vi "Configure All.vi"(1 "RT Data in":T1={"Device ref"=0, "Scan Period (uSec)"=10000, "Device Channels"={"Status"={"BD Refs"=[], "Length"=0, "FIFO Index"=0, "Data"=[]}, "Command"={"BD Refs"=[], "Data"=[], "Length"=0, "FIFO Index"=0}}, "Local Chassis"=[], "EtherCAT Masters"=[], "Async"={"Status"=refnum, "Command"=refnum, "Input FIFO"=refnum, "Input FIFO buffer"=[], "Output FIFO"=refnum, "Output FIFO buffer"=[], "Async VI Ref"=refnum}, "ECAT Reconfig"={"Reconfig Module Found"=FALSE, "VI Ref"=refnum, "Status"=refnum}, "Device Error"={"status"=FALSE, "code"=0, "source"=""}, "DeviceName"="", "PCLSync?"=FALSE} {"Device Channels"."Status"."BD Refs"."Data Reference" format="%.0x"; "Device Channels"."Command"."BD Refs"."Data Reference" format="%.0x"; "Local Chassis"."FPGA"."VS ref" format="%.0x"; "Local Chassis"."RSI Modules"."VS ref" format="%.0x"; "Local Chassis"."VS ref" format="%.0x"; "Device ref" format="%.0x"; "EtherCAT Masters"."REM IO ECAT Slaves"."VS ref" format="%.0x"; "EtherCAT Masters"."Generic EtherCAT Slaves"."VS ref" format="%.0x"; "EtherCAT Masters"."VS ref" format="%.0x"; "EtherCAT Masters"."EtherCAT Slaves"."FPGA"."VS ref" format="%.0x"; "EtherCAT Masters"."EtherCAT Slaves"."RSI Modules"."VS ref" format="%.0x"; "EtherCAT Masters"."EtherCAT Slaves"."VS ref" format="%.0x"}) -> (0 "RT Data out":T1={"Device ref"=0, "Scan Period (uSec)"=10000, "Device Channels"={"Status"={"BD Refs"=[], "Length"=0, "FIFO Index"=0, "Data"=[]}, "Command"={"BD Refs"=[], "Data"=[], "Length"=0, "FIFO Index"=0}}, "Local Chassis"=[], "EtherCAT Masters"=[], "Async"={"Status"=refnum, "Command"=refnum, "Input FIFO"=refnum, "Input FIFO buffer"=[], "Output FIFO"=refnum, "Output FIFO buffer"=[], "Async VI Ref"=refnum}, "ECAT Reconfig"={"Reconfig Module Found"=FALSE, "VI Ref"=refnum, "Status"=refnum}, "Device Error"={"status"=FALSE, "code"=0, "source"=""}, "DeviceName"="", "PCLSync?"=FALSE} {"Device Channels"."Status"."BD Refs"."Data Reference" format="%.0x"; "Device Channels"."Command"."BD Refs"."Data Reference" format="%.0x"; "Local Chassis"."FPGA"."VS ref" format="%.0x"; "Local Chassis"."RSI Modules"."VS ref" format="%.0x"; "Local Chassis"."VS ref" format="%.0x"; "Device ref" format="%.0x"; "EtherCAT Masters"."REM IO ECAT Slaves"."VS ref" format="%.0x"; "EtherCAT Masters"."Generic EtherCAT Slaves"."VS ref" format="%.0x"; "EtherCAT Masters"."VS ref" format="%.0x"; "EtherCAT Masters"."EtherCAT Slaves"."FPGA"."VS ref" format="%.0x"; "EtherCAT Masters"."EtherCAT Slaves"."RSI Modules"."VS ref" format="%.0x"; "EtherCAT Masters"."EtherCAT Slaves"."VS ref" format="%.0x"})   [LabVIEW 2020, in "SEECD Engine.lvlib"]
uses:
  SEECD Engine.lvlib
  Type Defs/RT Data.ctl
  <vilib>/NI VeriStand/Custom Device API/Custom Device Item Ref.ctl
  Type Defs/Device Channels.ctl
  Type Defs/Output Data.ctl
  <vilib>/NI VeriStand/Custom Device API/Block Data Reference.ctl
  <vilib>/NI VeriStand/Custom Device API/Data Reference.ctl
  Type Defs/Input Data.ctl
  Type Defs/Local Chassis Data.ctl
  Type Defs/RSI Module Data.ctl
  Type Defs/Open Module IOVs.ctl
  Includes/Modules.lvlibp/RSI Module/RSI Module.lvclass
  Includes/Modules.lvlibp/RSI Module/Module Models.ctl
  Includes/Modules.lvlibp/RSI Module/Channel Type.ctl
  Type Defs/Module Config Data.ctl
  Type Defs/Mixed IO.ctl
  Type Defs/FPGA Data.ctl
  Type Defs/UDV Data.ctl
  Shared/Type Defs/UDV Data Type.ctl
  Shared/Type Defs/FXP Config.ctl
  Type Defs/Mod Size Indexes.ctl
  Type Defs/EtherCAT Master Data.ctl
  Type Defs/EtherCAT Slave Data.ctl
  Type Defs/Generic ECAT Slave RT-Data-Array.ctl
  Type Defs/Generic ECAT Slave Data Cluster.ctl
  Type Defs/Generic ECAT Slave IOV Cluster.ctl
  Type Defs/REM IO ECAT Slave RT-Data-Array.ctl
  Type Defs/REM IO ECAT Slave Data Cluster.ctl
  Type Defs/REM IO ECAT Slave IOV Cluster.ctl
  Type Defs/Async Data.ctl
  Type Defs/Async Status.ctl
  Type Defs/Async State.ctl
  Type Defs/Async Command.ctl
  Type Defs/ECAT Reconfig Data.ctl
  Type Defs/ECAT Reconfig Status.ctl
  Type Defs/ECAT Reconfig State.ctl
  Type Defs/ECAT Module Reconfig.ctl
  <vilib>/NI VeriStand/Custom Device Tools/Custom Device Utility Library/Custom Device Utility Library.lvlib
  <resource>/objmgr/IndComECAT.rc
  <vilib>/NI VeriStand/Custom Device API/Custom Device API.lvlib
  Shared/SEECD Shared.lvlib
types:
  T1 = typedef "SEECD Engine.lvlib/RT Data.ctl" = cluster{"Device ref":T2, "Scan Period (uSec)":u32, "Device Channels":T3, "Local Chassis":T8[], "EtherCAT Masters":T20[], "Async":T28, "ECAT Reconfig":T29, "Device Error":errorcluster, "DeviceName":string, "PCLSync?":bool}
  T2 = typedef "Custom Device API.lvlib/Custom Device Item Ref.ctl" = u64
  T3 = typedef "SEECD Engine.lvlib/Device Channels.ctl" = cluster{"Status":T4, "Command":T7}
  T4 = typedef "SEECD Engine.lvlib/Output Data.ctl" = cluster{"BD Refs":T5[], "Length":i32, "FIFO Index":i32, "Data":dbl[]}
  T5 = typedef "Custom Device API.lvlib/Block Data Reference.ctl" = cluster{"Data Reference":T6, "Offset":u64, "Length":u64}
  T6 = typedef "Custom Device API.lvlib/Data Reference.ctl" = i32
  T7 = typedef "SEECD Engine.lvlib/Input Data.ctl" = cluster{"BD Refs":T5[], "Data":dbl[], "Length":i32, "FIFO Index":i32}
  T8 = typedef "SEECD Engine.lvlib/Local Chassis Data.ctl" = cluster{"VS ref":T2, "RSI Modules":T9[], "FPGA":T15[], "Input Mod Size Idxs":T19, "Output Modules":i32[], "MixedIO Mod Size Idxs":T19}
  T9 = typedef "SEECD Engine.lvlib/RSI Module Data.ctl" = cluster{"VS ref":T2, "IOV ref":refnum<k21>, "Open Mod refs":T10, "Module DVR":refnum<data-value>, "Slot":u32, "Model":T11, "Channel Type":T12, "EtherCAT?":bool, "CDInput Data":T7, "CDOutput Data":T4, "Module Config Data":T13, "Mixed IO":T14}
  T10 = typedef "SEECD Engine.lvlib/Open Module IOVs.ctl" = cluster{"Analog Read":refnum<k21>, "Digital Read":refnum<k21>, "Analog Write":refnum<k21>, "Digital Write":refnum<k21>}
  T11 = typedef "Modules.lvlibp/RSI Module.lvclass/Module Models.ctl" = enum16{"Empty", "NI 9201", "NI 9203", "NI 9205", "NI 9206", "NI 9207", "NI 9208", "NI 9209", "NI 9210", "NI 9211", "NI 9212", "NI 9213", "NI 9214", "NI 9215", "NI 9216", "NI 9217", "NI 9219", "NI 9220", "NI 9221", "NI 9222", "NI 9223", "NI 9224", "NI 9225", "NI 9226", "NI 9227", "NI 9228", "NI 9229", "NI 9233", "NI 9234", "NI 9235", "NI 9236", "NI 9237", "NI 9239", "NI 9242", "NI 9244", "NI 9253", "NI 9263", "NI 9264", "NI 9265", "NI 9266", "NI 9269", "NI 9344", "NI 9350", "NI 9375", "NI 9401", "NI 9402", "NI 9403", "NI 9411", "NI 9421", "NI 9422", "NI 9423", "NI 9425", "NI 9426", "NI 9435", "NI 9436", "NI 9437", "NI 9472", "NI 9474", "NI 9475", "NI 9476", "NI 9477", "NI 9478", "NI 9481", "NI 9482", "NI 9485"}
  T12 = typedef "Modules.lvlibp/RSI Module.lvclass/Channel Type.ctl" = enum16{"Analog", "Digital"}
  T13 = typedef "SEECD Engine.lvlib/Module Config Data.ctl" = cluster{"Configurable?":bool, "Config Block Data Refs":T5[], "Config Data DVR":refnum<data-value>, "Previous Values":dbl[], "Local Reconfig VI Ref":refnum<vi>}
  T14 = typedef "SEECD Engine.lvlib/Mixed IO.ctl" = cluster{"Input Channel Indices":i32[], "Input Buffer":dbl[]}
  T15 = typedef "SEECD Engine.lvlib/FPGA Data.ctl" = cluster{"VS ref":T2, "IOV ref":refnum<k21>, "FPGA Target":enum16{"Local", "EtherCAT"}, "Product Code":u32, "Bitfile Signature":string, "Bitfile Path (RT)":path, "FPGA Session":u32, "Input Data":T7, "Output Data":T4, "UDVs":cluster{"From FPGA":T16[], "To FPGA":T16[]}}
  T16 = typedef "SEECD Engine.lvlib/UDV Data.ctl" = cluster{"VS ref":T2, "IOV Ref":refnum<k21>, "Name":string, "UDV Data Type":T17, "Supported Type?":bool, "FXP Config":T18, "FXP VI Ref":refnum<vi>}
  T17 = typedef "SEECD Shared.lvlib/UDV Data Type.ctl" = enum16{"Boolean", "Fixed Point", "Int8", "Int16", "Int32", "Int64", "U32 Bit Field", "UInt8", "UInt16", "UInt32", "UInt64", "Other", "DBL", "SGL"}
  T18 = typedef "SEECD Shared.lvlib/FXP Config.ctl" = cluster{"signed":bool, "size":u32, "integersize":i32}
  T19 = typedef "SEECD Engine.lvlib/Mod Size Indexes.ctl" = cluster{"4":i32[], "8":i32[], "16":i32[], "32":i32[], "other":i32[]}
  T20 = typedef "SEECD Engine.lvlib/EtherCAT Master Data.ctl" = cluster{"VS ref":T2, "IOV ref":refnum<k21>, "Master ID":u32, "Cyclic Data Bandwidth":u32, "EtherCAT Slaves":T21[], "Generic EtherCAT Slaves":T22, "REM IO ECAT Slaves":T25}
  T21 = typedef "SEECD Engine.lvlib/EtherCAT Slave Data.ctl" = cluster{"VS ref":T2, "IOV ref":refnum<k21>, "Position Address":u16, "RSI Modules":T9[], "FPGA":T15[], "Input Mod Size Idxs":T19, "Output Modules":i32[], "MixedIO Mod Size Idxs":T19}
  T22 = typedef "SEECD Engine.lvlib/Generic ECAT Slave RT-Data-Array.ctl" = T23[]
  T23 = typedef "SEECD Engine.lvlib/Generic ECAT Slave Data Cluster.ctl" = cluster{"VS ref":T2, "IOV ref":refnum<k21>, "Position Address":u16, "I/O Imput Vars ":T24[], "I/O Output Vars":T24[], "I/O Input Data":T7, "I/O Output Data":T4, "Distributed Clock":bool}
  T24 = typedef "SEECD Engine.lvlib/Generic ECAT Slave IOV Cluster.ctl" = cluster{"VS ref":T2, "IOV Ref":refnum<k21>, "Name":string, "UDV Data Type":T17}
  T25 = typedef "SEECD Engine.lvlib/REM IO ECAT Slave RT-Data-Array.ctl" = T26[]
  T26 = typedef "SEECD Engine.lvlib/REM IO ECAT Slave Data Cluster.ctl" = cluster{"VS ref":T2, "IOV ref":refnum<k21>, "Position Address":u16, "I/O Imput Vars ":T27[], "I/O Output Vars":T27[], "I/O Input Data":T7, "I/O Output Data":T4}
  T27 = typedef "SEECD Engine.lvlib/REM IO ECAT Slave IOV Cluster.ctl" = cluster{"VS ref":T2, "IOV Ref":refnum<k21>, "Name":string, "UDV Data Type":T17, "Scaling Factor":dbl}
  T28 = typedef "SEECD Engine.lvlib/Async Data.ctl" = cluster{"Status":refnum<queue>, "Command":refnum<queue>, "Input FIFO":refnum<k33>, "Input FIFO buffer":dbl[], "Output FIFO":refnum<k33>, "Output FIFO buffer":dbl[], "Async VI Ref":refnum<vi>}
  T29 = typedef "SEECD Engine.lvlib/ECAT Reconfig Data.ctl" = cluster{"Reconfig Module Found":bool, "VI Ref":refnum<vi>, "Status":refnum<queue>}
  T30 = typedef "SEECD Engine.lvlib/ECAT Module Reconfig.ctl" = cluster{"Module DVR":refnum<data-value>, "IOV ref":refnum<k21>, "Config Data DVR":refnum<data-value>}
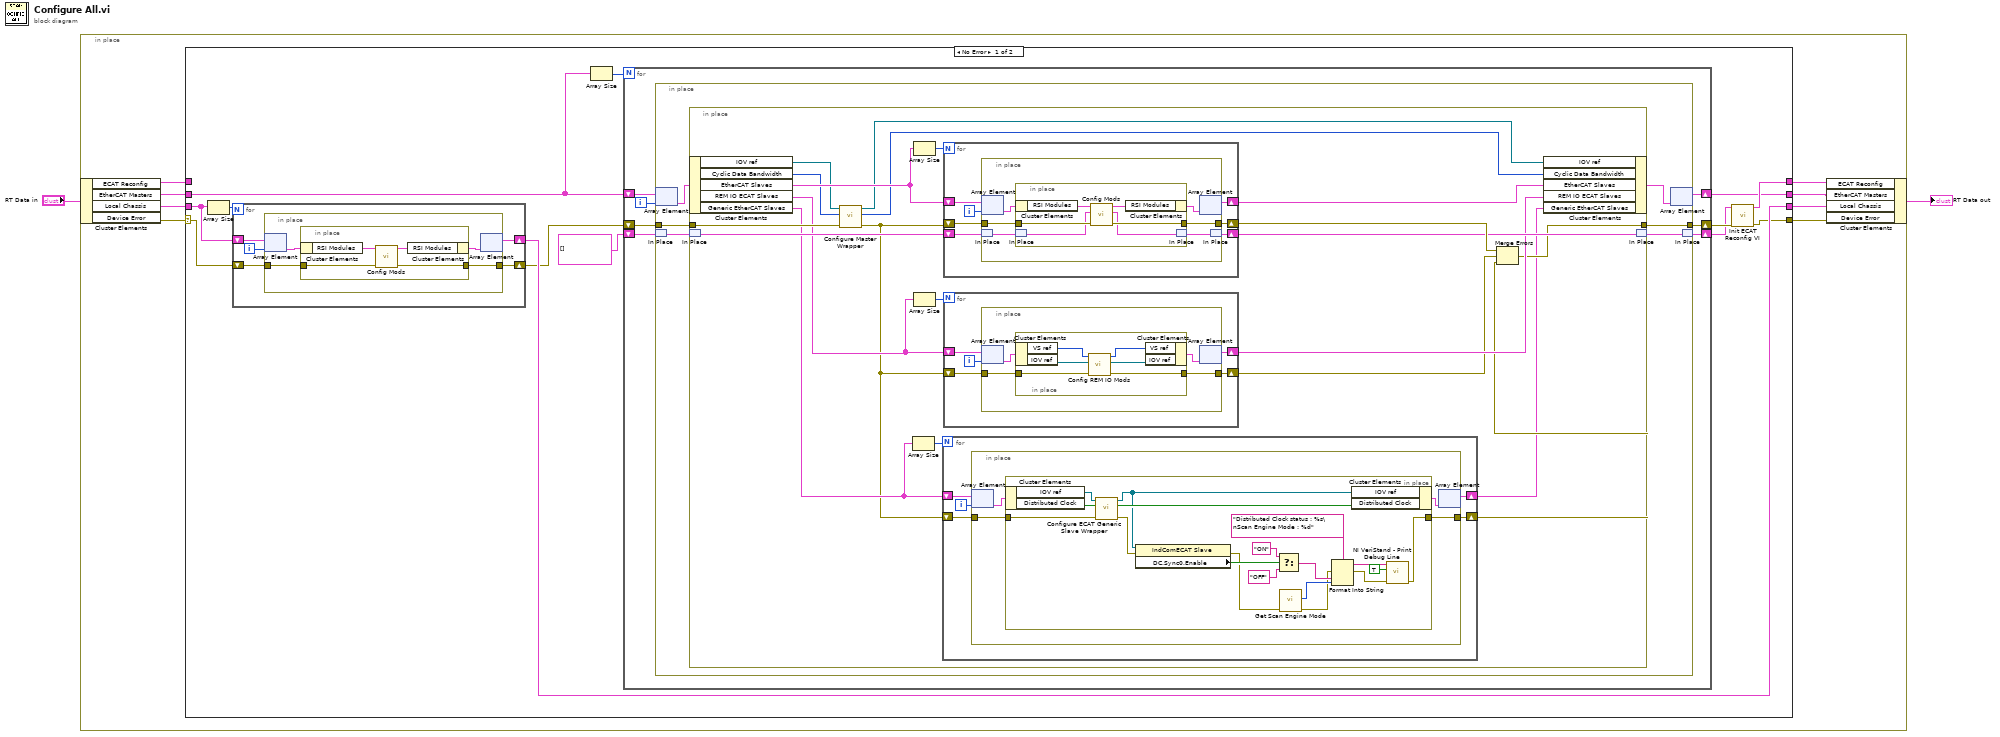
[diagram p0: block diagram]
diagram:
  n1 = in-place {
    n2 = in-place-cluster #1("RT Data in") -> ("ECAT Reconfig"=w3:T29, "EtherCAT Masters"=w9:T20[], "Local Chassis"=w8:T8[], "Device Error"=w10:errorcluster)
    n3 = case shown="No Error" w10 {
      selector: w10 -> [w19 w135]
      tunnel: [w12 w135] -> w7
      tunnel: w9 -> [w22 w133]
      tunnel: w8 -> [w20 w134]
      tunnel: [w18 w134] -> w6
      tunnel: [w11 w133] -> w5
      tunnel: [w13 w132] -> w4
      tunnel: w3 -> [_ w132]
      frame No Error {
        n4 = Array Size(array=w20) -> (size(s)=w21:i32)
        n5 = for {
          N: w21 -> [_]
          shift-right: [w24] -> w18
          shift-left: w20 -> [w28]
          shift-right: [w25] -> w17
          shift-left: w19 -> [w26]
          i -> [w27]
          n6 = in-place {
            in-place-border: w26 -> [w30]
            in-place-border: [w29] -> w25
            n7 = in-place-array #2(w28, w27) -> (w32:T8)
            n8 = in-place {
              in-place-border: w30 -> [w34]
              in-place-border: [w33] -> w29
              n9 = in-place-cluster #3(w32) -> ("RSI Modules"=w36:T9[])
              n10 = call "Config Mods.vi"("error in (no error)"=w34, "RSI Modules in"=w36) -> ("error out"=w33:errorcluster, "RSI Modules out"=w35:T9[])  [unwired: 7 in, 1 out]
              n11 = in-place-cluster #3("RSI Modules"=w35) -> (w31:T8)
            }
            n12 = in-place-array #2(w31) -> (w24:T8[])  [unwired: 1 out]
          }
        }
        n13 = Array Size(array=w22) -> (size(s)=w23:i32)
        n14 = for {
          N: w23 -> [_]
          shift-right: [w40] -> w15
          shift-left: w17 -> [w41]
          shift-right: [w39] -> w11
          shift-left: w22 -> [w43]
          shift-right: [w37] -> w14
          shift-left: T30[] [] -> [w38]
          i -> [w42]
          n15 = in-place {
            in-place-border: w41 -> [w48]
            in-place-border: [w47] -> w40
            n16 = in-place-array #4(w43, w42) -> (w49:T20)
            n17 = in-place-match #5(w38) -> (w45:T30[])
            n18 = in-place {
              in-place-border: w48 -> [w64]
              in-place-border: [w56] -> w47
              n19 = in-place-cluster #6(w49) -> ("IOV ref"=w62:refnum<k21>, "Cyclic Data Bandwidth"=w63:u32, "EtherCAT Slaves"=w70:T21[], "REM IO ECAT Slaves"=w59:T25, "Generic EtherCAT Slaves"=w53:T22)
              n20 = in-place-match #7(w45) -> (w66:T30[])
              n21 = call "Configure Master Wrapper.vi"("error in"=w64, "Cyclic Data Bandwidth"=w63, "IOV ref in"=w62) -> ("error out"=w50:errorcluster, "Cyclic Data Bandwidth out"=w61:u32, "IOV ref out"=w60:refnum<k21>)  [unwired: 6 in]
              n22 = Array Size(array=w53) -> (size(s)=w54:i32)
              n23 = Array Size(array=w70) -> (size(s)=w69:i32)
              n24 = Array Size(array=w59) -> (size(s)=w57:i32)
              n25 = for {
                N: w54 -> [_]
                shift-right: [w71] -> w52
                shift-left: w50 -> [w74]
                shift-right: [w73] -> w51
                shift-left: w53 -> [w72]
                i -> [w75]
                n26 = in-place {
                  in-place-border: w74 -> [w79]
                  in-place-border: [w78] -> w71
                  n27 = in-place-array #8(w72, w75) -> (w76:T23)
                  n28 = in-place {
                    in-place-border: w79 -> [w97]
                    in-place-border: [w92] -> w78
                    n29 = in-place-cluster #9(w76) -> ("IOV ref"=w94:refnum<k21>, "Distributed Clock"=w96:bool)
                    n30 = call "Configure ECAT Generic Slave Wrapper.vi"("error in"=w97, "Distributed Clock"=w96, "IOV ref"=w94) -> ("error out"=w93:errorcluster, "Distributed Clock out"=w95:bool, "IOV ref out"=w91:refnum<k21>)  [unwired: 6 in]
                    n31 = property class="IndComECAT Slave"(reference=w91, error in=w93) -> (error out=w82:errorcluster, "DC.Sync0.Enable"=w86:bool)  [unwired: 1 out]
                    n32 = Select(t="ON" ("format string"), s=w86, f="OFF" ("format string")) -> (s? t:f=w84:string)
                    n33 = call <vilib>:"Get Scan Engine Mode.vi"("error in (no error)"=w82) -> ("error out"=w80:errorcluster, "mode"=w81:i32)  [unwired: 9 in]
                    n34 = Format Into String(format string="Distributed Clock status : %s\nScan Engine Mode : %d", error in=w80, w84, w81) -> (resulting string=w90:string, error out=w88:errorcluster)  [unwired: 1 in]
                    n35 = in-place-cluster #9("IOV ref"=w91, "Distributed Clock"=w95) -> (w77:T23)
                    n36 = call <vilib>:"NI VeriStand - Print Debug Line.vi"("error in (no error)"=w88, "Add to log file? (F)"=TRUE, "Message"=w90) -> ("error out"=w92:errorcluster)  [unwired: 8 in]
                  }
                  n37 = in-place-array #8(w77) -> (w73:T22)  [unwired: 1 out]
                }
              }
              n38 = for {
                N: w69 -> [_]
                shift-right: [w116] -> w68
                shift-left: w50 -> [w117]
                shift-right: [w115] -> w67
                shift-left: w70 -> [w119]
                shift-right: [w113] -> w65
                shift-left: w66 -> [w114]
                i -> [w118]
                n39 = in-place {
                  in-place-border: w117 -> [w124]
                  in-place-border: [w123] -> w116
                  n40 = in-place-array #10(w119, w118) -> (w125:T21)
                  n41 = in-place-match #11(w114) -> (w121:T30[])
                  n42 = in-place {
                    in-place-border: w124 -> [w129]
                    in-place-border: [w128] -> w123
                    n43 = in-place-cluster #12(w125) -> ("RSI Modules"=w131:T9[])
                    n44 = in-place-match #13(w121) -> (w127:T30[])
                    n45 = call "Config Mods.vi"("error in (no error)"=w129, "ECAT Mod Reconfig in"=w127, "RSI Modules in"=w131) -> ("error out"=w128:errorcluster, "ECAT Mod Reconfig out"=w126:T30[], "RSI Modules out"=w130:T9[])  [unwired: 6 in]
                    n46 = in-place-cluster #12("RSI Modules"=w130) -> (w122:T21)
                    n47 = in-place-match #13(w126) -> (w120:T30[])
                  }
                  n48 = in-place-array #10(w122) -> (w115:T21[])  [unwired: 1 out]
                  n49 = in-place-match #11(w120) -> (w113:T30[])
                }
              }
              n50 = for {
                N: w57 -> [_]
                shift-right: [w98] -> w55
                shift-left: w50 -> [w101]
                shift-right: [w100] -> w58
                shift-left: w59 -> [w99]
                i -> [w102]
                n51 = in-place {
                  in-place-border: w101 -> [w106]
                  in-place-border: [w103] -> w98
                  n52 = in-place-array #14(w99, w102) -> (w105:T26)
                  n53 = in-place {
                    in-place-border: w106 -> [w112]
                    in-place-border: [w111] -> w103
                    n54 = in-place-cluster #15(w105) -> ("VS ref"=w108:T2, "IOV ref"=w110:refnum<k21>)
                    n55 = call "Config REM IO Mods.vi"("error in (no error)"=w112, "IOV Ref In"=w110, "VS Ref In"=w108) -> ("error out"=w111:errorcluster, "IOV Ref Out"=w109:refnum<k21>, "VS Ref Out"=w107:T2)  [unwired: 6 in]
                    n56 = in-place-cluster #15("VS ref"=w107, "IOV ref"=w109) -> (w104:T26)
                  }
                  n57 = in-place-array #14(w104) -> (w100:T25)  [unwired: 1 out]
                }
              }
              n58 = Merge Errors(w68, w55, w52) -> (w56:errorcluster)
              n59 = in-place-cluster #6("IOV ref"=w60, "Cyclic Data Bandwidth"=w61, "EtherCAT Slaves"=w67, "REM IO ECAT Slaves"=w58, "Generic EtherCAT Slaves"=w51) -> (w46:T20)
              n60 = in-place-match #7(w65) -> (w44:T30[])
            }
            n61 = in-place-array #4(w46) -> (w39:T20[])  [unwired: 1 out]
            n62 = in-place-match #5(w44) -> (w37:T30[])
          }
        }
        n63 = call "Init ECAT Reconfig VI.vi"("error in (no error)"=w15, "ECAT Modules"=w14) -> ("error out"=w12:errorcluster, "ECAT Reconfig out"=w13:T29)  [unwired: 8 in]
      }
      frame Error {
      }
    }
    n64 = in-place-cluster #1("ECAT Reconfig"=w4, "EtherCAT Masters"=w5, "Local Chassis"=w6, "Device Error"=w7) -> (→"RT Data out":T1)
  }
